vi "calculate_header_width.vi"(8 "error in (no error)":errorcluster, 11 "listbox_reference":refnum<vi>) -> (0 "error out":errorcluster, 4 "width []":u32[](array[numeric]), 6 "height []":u32[](array[numeric]))   [LabVIEW 2015, in "lv-pagination.lvlib"]
uses:
  lv-pagination.lvlib
  <vilib>/Utility/miscctls.llb/LVRowAndColumnTypeDef.ctl
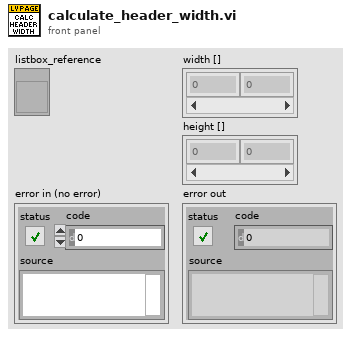
[diagram p1: front panel]
types:
  T1 = enum16{"User-specified Font", "Application Font", "System Font", "Dialog Font"}
  T2 = typedef "LVRowAndColumnTypeDef.ctl" = cluster{"Row":i32, "Column":i32}
  T3 = cluster{"CellFontName":string, "CellFontSize":u32, "CellFontStrike":bool, "CellFontItalic":bool, "CellFontUnder":bool, bool, bool, "CellFontBold":bool}
  T4 = cluster{"left":i16, "top":i16, "right":i16, "bottom":i16}
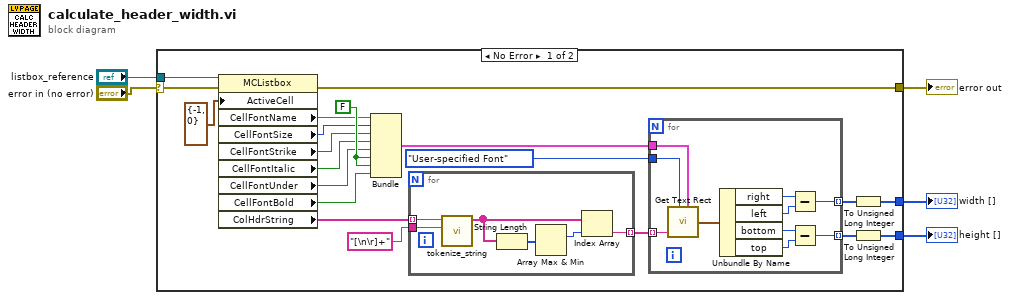
[diagram p0: block diagram]
diagram:
  n1 = case shown="No Error" "error in (no error)" {
    selector: "error in (no error)" -> [w14 w42]
    tunnel: "listbox_reference" -> [w15 _]
    tunnel: [w12 w42] -> w3
    tunnel: [w7 _] -> w2
    tunnel: [w6 _] -> w1
    frame No Error {
      w23 = FALSE
      n2 = property on="Property Node" class="MCListbox"(reference=w15, error in=w14, "ActiveCell"=T2 {"Row"=-1, "Column"=0} ("Active Cell:Active Cell")) -> (error out=w12:errorcluster, "CellFontName"=w17:string, "CellFontSize"=w18:u32, "CellFontStrike"=w19:bool, "CellFontItalic"=w20:bool, "CellFontUnder"=w21:bool, "CellFontBold"=w22:bool, "ColHdrString"=w13:string[])  [unwired: 1 out]
      n3 = Bundle("CellFontName"=w17, "CellFontSize"=w18, "CellFontStrike"=w19, "CellFontItalic"=w20, "CellFontUnder"=w21, w23, w23, "CellFontBold"=w22) -> (w11:T3)  [unwired: 1 in]
      n4 = for {
        tunnel: w13 -> [w27] mode=indexing
        tunnel: [w29] -> w25 mode=indexing
        tunnel: "[\n\r]+" ("delimiter ([\\s\\t\\n\\r]+)") -> [w26]
        n5 = call "tokenize_string.vi"("delimiter"=w26, "input_string"=w27) -> ("delimited_string []"=w28:string[])  [unwired: 8 in, 1 out]
        n6 = String Length(string=w28) -> (length=w30:i32[])
        n7 = Array Max & Min(array=w30) -> (max index (indices)=w31:i32)  [unwired: 3 out]
        n8 = Index Array(array=w28, index=w31) -> (element=w29:string)
      }
      n9 = for {
        tunnel: w25 -> [w38] mode=indexing
        tunnel: w11 -> [w37]
        tunnel: [w36] -> w9 mode=indexing
        tunnel: T1."User-specified Font" ("desired font(Application)") -> [w35]
        tunnel: [w32] -> w8 mode=indexing
        n10 = call <vilib>:"Get Text Rect.vi"("desired font(Application)"=w35, "text"=w38, "[user-specified font]"=w37) -> ("rect"=w41:T4)  [unwired: 6 in]
        n11 = Unbundle By Name(w41) -> ("right"=w40:i16, "left"=w39:i16, "bottom"=w34:i16, "top"=w33:i16)
        n12 = Subtract(x=w40, y=w39) -> (x-y=w36:i16)
        n13 = Subtract(x=w34, y=w33) -> (x-y=w32:i16)
      }
      n14 = To Unsigned Long Integer(number=w9) -> (unsigned 32bit integer=w7:u32[])
      n15 = To Unsigned Long Integer(number=w8) -> (unsigned 32bit integer=w6:u32[])
    }
    frame Error {
    }
  }
  "error out" <- w3
  "width []" <- w2
  "height []" <- w1
